vi "AutoDriveShoot.vi"(6 "Reset?":bool, 7 "Drive Params":T1, 8 "Drive PID":T2={"X Dist"={"PID gains"={"proportional gain (Kc)"=1.0, "integral time (Ti, min)"=0.0, "derivative time (Td, min)"=0.0}, "output range"={"output high"=1.0, "output low"=-1.0}}, "Y Dist"={"PID gains"={"proportional gain (Kc)"=1.0, "integral time (Ti, min)"=0.0, "derivative time (Td, min)"=0.0}, "output range"={"output high"=1.0, "output low"=-1.0}}} {"Y Dist"."output range"."output low" format="%.2f"; "Y Dist"."output range"."output high" format="%.2f"; "Y Dist"."PID gains"."derivative time (Td, min)" format="%.3f"; "Y Dist"."PID gains"."integral time (Ti, min)" format="%.3f"; "Y Dist"."PID gains"."proportional gain (Kc)" format="%.3f"; "X Dist"."output range"."output low" format="%.2f"; "X Dist"."output range"."output high" format="%.2f"; "X Dist"."PID gains"."derivative time (Td, min)" format="%.3f"; "X Dist"."PID gains"."integral time (Ti, min)" format="%.3f"; "X Dist"."PID gains"."proportional gain (Kc)" format="%.3f"}, 11 "Array":dbl[](array[numeric]) format="%0.3f") -> (3 "Finished":bool)   [LabVIEW 2013]
uses:
  AutoDriveParams.ctl
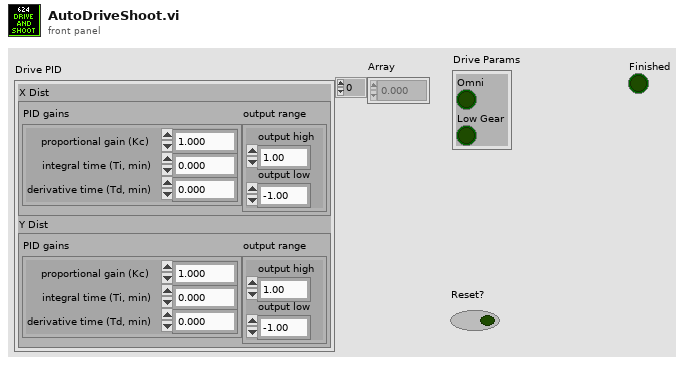
[diagram p1: front panel]
types:
  T1 = typedef "AutoDriveParams.ctl" = cluster{"Omni":bool, "Low Gear":bool}
  T2 = cluster{"X Dist":cluster{"PID gains":cluster{"proportional gain (Kc)":dbl, "integral time (Ti, min)":dbl, "derivative time (Td, min)":dbl}, "output range":cluster{"output high":dbl, "output low":dbl}}, "Y Dist":cluster{"PID gains":cluster{"proportional gain (Kc)":dbl, "integral time (Ti, min)":dbl, "derivative time (Td, min)":dbl}, "output range":cluster{"output high":dbl, "output low":dbl}}}
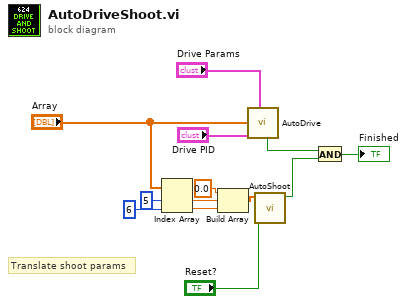
[diagram p0: block diagram]
diagram:
  # "Translate shoot params"
  n1 = Index Array(array="Array", index #1=5 ("index"), index #2=6 ("index")) -> (element #1=w9:dbl, element #2=w1:dbl)
  n2 = Build Array(0.0 ("element"), w9, w1) -> (w4:dbl[])
  n3 = call "AutoDrive.vi"("Drive Params"="Drive Params", "Drive PID"="Drive PID", "Array"="Array") -> ("isFinished"=w13:bool)  [unwired: 8 in]
  n4 = call "AutoShoot.vi"("Reset?"="Reset?", "Array"=w4) -> ("isFinished"=w12:bool)  [unwired: 9 in]
  n5 = And(x=w13, y=w12) -> (x .and. y?=→"Finished":bool)
